vi "MH_DataToPTUTag.vi"(8 "error in":errorcluster, 10 "TagIn":T1) -> (0 "error in 2":errorcluster, 1 "AuxStrTagValue":string, 2 "TagValue":i64, 3 "TagIdent Out":string, 4 "StrTagType":string)   [LabVIEW 2019]
uses:
  <vilib>/Utility/miscctls.llb/LVDateTimeRec.ctl
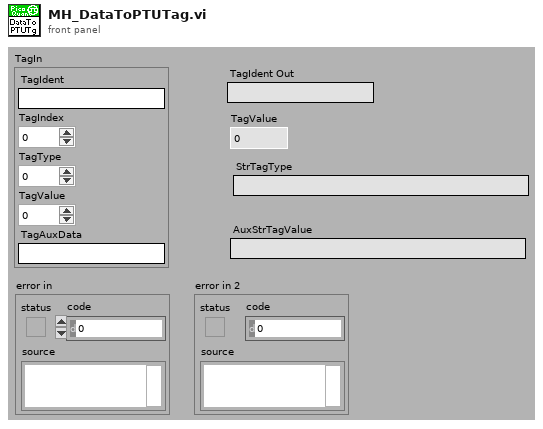
[diagram p1: front panel]
types:
  T1 = cluster{"TagIdent":string, "TagIndex":i32, "TagType":i32, "TagValue":i64, "TagAuxData":string}
  T2 = cluster{"File_GUID":string, "File_AssuredContent":string, "CreatorSW_ContentVersion":string, "CreatorSW_Name":string, "CreatorSW_Version":string, "horodatage":timestamp, "File_Comment":string}
  T3 = typedef "LVDateTimeRec.ctl" = cluster{"fractional second":dbl, "second":i32, "minute":i32, "hour":i32, "day of month":i32, "month":i32, "year":i32, "day of week":i32, "day of year":i32, "DST":i32}
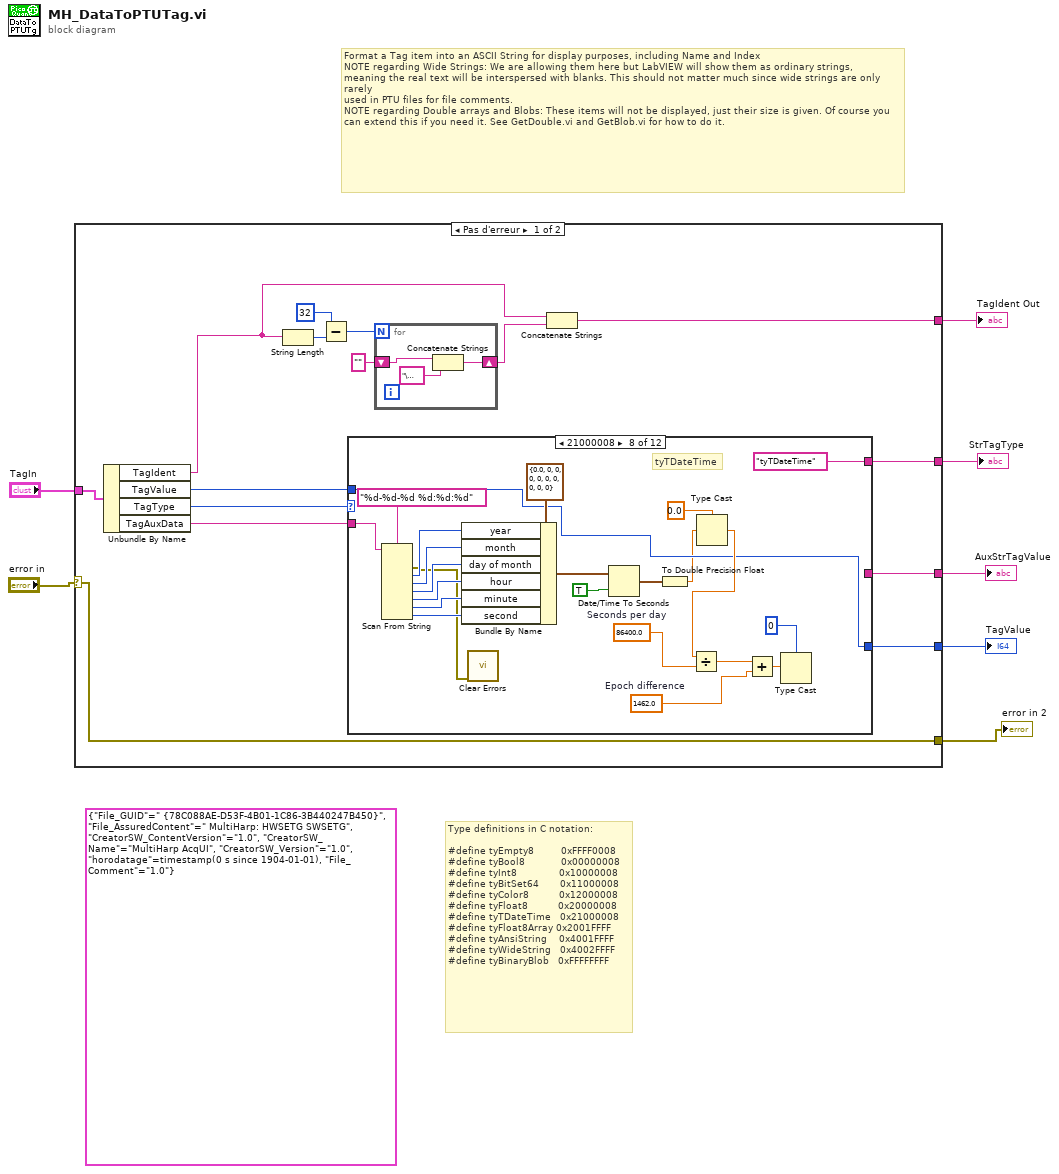
[diagram p0: block diagram]
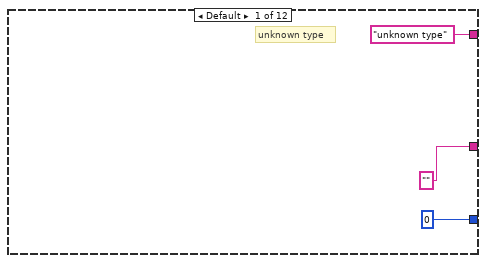
[diagram p2: hidden frame]
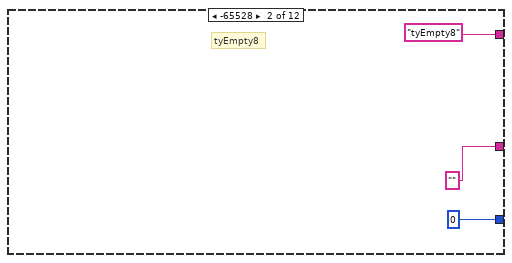
[diagram p3: hidden frame]
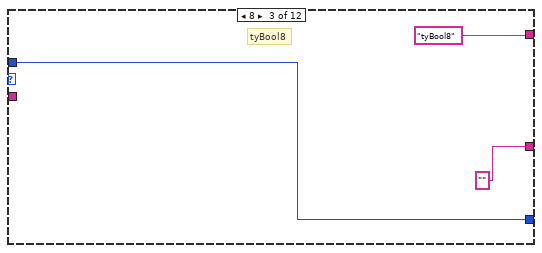
[diagram p4: hidden frame]
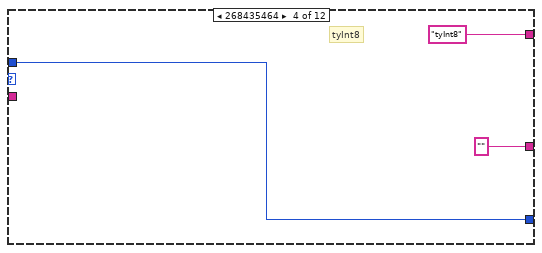
[diagram p5: hidden frame]
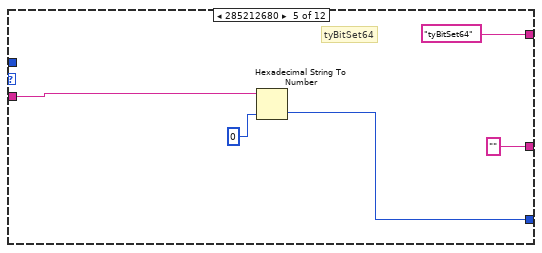
[diagram p6: hidden frame]
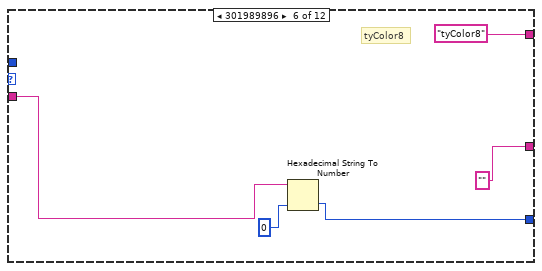
[diagram p7: hidden frame]
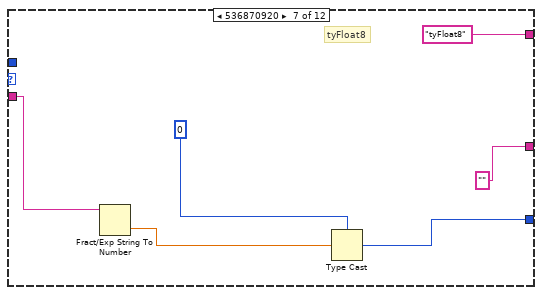
[diagram p8: hidden frame]
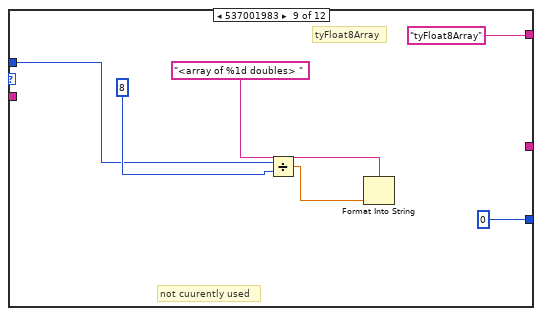
[diagram p9: hidden frame]
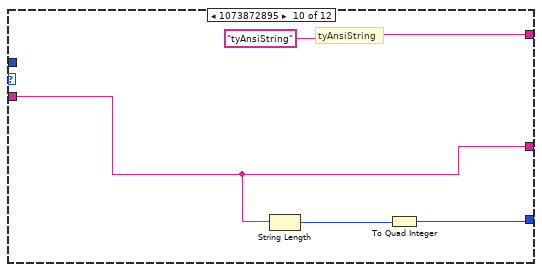
[diagram p10: hidden frame]
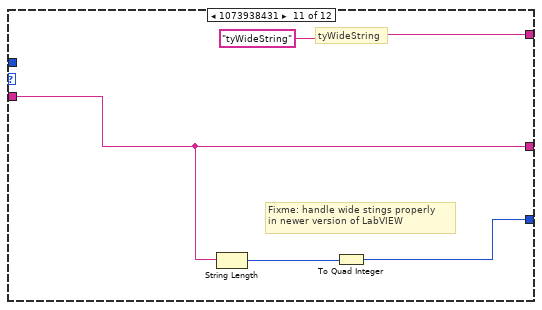
[diagram p11: hidden frame]
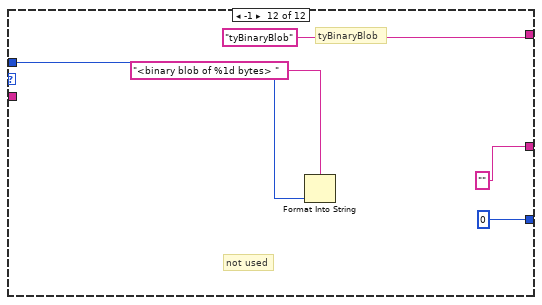
[diagram p12: hidden frame]
diagram:
  (unwired) T2 {"File_GUID"=" {78C088AE-D53F-4B01-1C86-3B440247B450}", "File_AssuredContent"=" MultiHarp: HWSETG SWSETG", "CreatorSW_ContentVersion"="1.0", "CreatorSW_Name"="MultiHarp AcqUI", "CreatorSW_Version"="1.0", "horodatage"=timestamp(0 s since 1904-01-01), "File_Comment"="1.0"}
  # "Type definitions in C notation:\n\n#define tyEmpty8         0xFFFF0008\n#define tyBool8            0x00000008\n#define tyInt8              0x10000008\n#define tyBitSet64       0x11000008\n#define tyColor8          0x12000008\n#define tyFloat8          0x20000008\n#define tyTDateTime   0x21000008\n#define tyFloat8Array 0x2001FFFF\n#define tyAnsiString    0x4001FFFF\n#define tyWideString   0x4002FFFF\n#define tyBinaryBlob   0xFFFFFFFF"
  # "Format a Tag item into an ASCII String for display purposes, including Name and Index\nNOTE regarding Wide Strings: We are allowing them here but LabVIEW will show them as ordinary strings, \nmeaning the real text will be interspersed with blanks. This should not matter much since wide strings are only rarely \nused in PTU files for file comments.\nNOTE regarding Double arrays and Blobs: These items will not be displayed, just their size is given. Of course you\ncan extend this if you need it. See GetDouble.vi and GetBlob.vi for how to do it."
  n1 = case shown="Pas d'erreur" "error in" {
    selector: "error in" -> [w10 w96]
    tunnel: [w22 _] -> w7
    tunnel: [w21 _] -> w6
    tunnel: [w16 _] -> w5
    tunnel: [w13 _] -> w4
    tunnel: "TagIn" -> [w12 _]
    tunnel: [w10 w96] -> w1
    frame No Error {
      n2 = Unbundle By Name(w12) -> ("TagIdent"=w11:string, "TagValue"=w14:i64, "TagType"=w9:i32, "TagAuxData"=w15:string)
      n3 = String Length(string=w11) -> (length=w20:i32)
      n4 = Subtract(x=32, y=w20) -> (x-y=w18:i32)
      n5 = case shown="21000008" w9 {
        tunnel: w14 -> [_ _ w32 w36 _ _ _ w55 w81 _ _ w93]
        tunnel: ["" ("TagAuxData") "" ("TagAuxData") "" ("TagAuxData") "" ("TagAuxData") "" ("TagAuxData") "" ("TagAuxData") "" ("TagAuxData") _ _ w85 w88 "" ("TagAuxData")] -> w21
        tunnel: w15 -> [_ _ _ _ w40 w45 w50 w60 _ w85 w88 _]
        tunnel: ["unknown type" ("string") "tyEmpty8" ("string") "tyBool8" ("string") "tyInt8" ("string") "tyBitSet64" ("string") "tyColor8" ("string") "tyFloat8" ("string") "tyTDateTime" ("string") "tyFloat8Array" ("string") "tyAnsiString" ("string") "tyWideString" ("string") "tyBinaryBlob" ("string")] -> w22
        tunnel: [i64 0 ("TagValue") i64 0 ("TagValue") w32 w36 w39 w44 w51 w55 i64 0 ("TagValue") w83 w87 i64 0 ("TagValue")] -> w13
        frame Default {
          # "unknown type"
        }
        frame -65528 {
          # "tyEmpty8"
        }
        frame 8 {
          # "tyBool8"
        }
        frame 268435464 {
          # "tyInt8"
        }
        frame 285212680 {
          # "tyBitSet64"
          n6 = Hexadecimal String To Number(string=w40, default (0uL)=i64 0 ("TagValue")) -> (number=w39:i64)  [unwired: 1 in, 1 out]
        }
        frame 301989896 {
          # "tyColor8"
          n7 = Hexadecimal String To Number(string=w45, default (0uL)=i64 0 ("TagValue")) -> (number=w44:i64)  [unwired: 1 in, 1 out]
        }
        frame 536870920 {
          # "tyFloat8"
          n8 = Fract/Exp String To Number(string=w50) -> (number=w49:dbl)  [unwired: 3 in, 1 out]
          n9 = Type Cast(type=i64 0 ("TagValue"), x=w49) -> (*(type *) &x=w51:i64)
        }
        frame 553648136 {
          w75 = 86400.0  # Seconds per day
          w73 = 1462.0  # Epoch difference
          # "tyTDateTime"
          n10 = Scan From String(format string="%d-%d-%d %d:%d:%d" ("chaîne de format"), input string=w60) -> (error out=w56:errorcluster, output 1=w63:i32, output 2=w64:i32, output 3=w65:i32, output 4=w66:i32, output 5=w67:i32, output 6=w68:i32)  [unwired: 8 in, 2 out]
          n11 = Bundle By Name(cluster=T3 {"fractional second"=0.0, "second"=0, "minute"=0, "hour"=0, "day of month"=0, "month"=0, "year"=0, "day of week"=0, "day of year"=0, "DST"=0} ("cluster date/heure"), "year"=w63, "month"=w64, "day of month"=w65, "hour"=w66, "minute"=w67, "second"=w68) -> (w62:T3)
          n12 = call <vilib>:"Clear Errors.vi"("error in (no error)"=w56) -> ()  [unwired: 5 in, 2 out]
          n13 = Date/Time To Seconds(1:TRUE ("UTC (F)"), 2:w62) -> (0:w59:timestamp)
          n14 = To Double Precision Float(number=w59) -> (double precision float=w54:dbl)
          n15 = Type Cast(type=0.0, x=w54) -> (*(type *) &x=w57:dbl)
          n16 = Divide(x=w57, y=w75) -> (x/y=w74:dbl)
          n17 = Add(x=w74, y=w73) -> (x+y=w72:dbl)
          n18 = Type Cast(type=i64 0 ("TagValue"), x=w72) -> ()  [unwired: 1 out]
        }
        frame 537001983 {
          # "not cuurently used"
          # "tyFloat8Array"
          n19 = Divide(x=w81, y=i64 8) -> (x/y=w80:dbl)
          n20 = Format Into String(format string="<array of %1d doubles> ", w80) -> ()  [unwired: 2 in, 2 out]
        }
        frame 1073872895 {
          # "tyAnsiString"
          n21 = String Length(string=w85) -> (length=w84:i32)
          n22 = To Quad Integer(1:w84) -> (0:w83:i64)
        }
        frame 1073938431 {
          # "Fixme: handle wide stings properly \nin newer version of LabVIEW"
          # "tyWideString"
          n23 = String Length(string=w88) -> (length=w89:i32)
          n24 = To Quad Integer(1:w89) -> (0:w87:i64)
        }
        frame -1 {
          # "not used"
          # "tyBinaryBlob"
          n25 = Format Into String(format string="<binary blob of %1d bytes> ", w93) -> ()  [unwired: 2 in, 2 out]
        }
      }
      n26 = for {
        N: w18 -> [_]
        shift-right: [w25] -> w17
        shift-left: "" -> [w24]
        n27 = Concatenate Strings(w24, "\u0000") -> (w25:string)
      }
      n28 = Concatenate Strings(w11, w17) -> (w16:string)
    }
    frame Error {
    }
  }
  "StrTagType" <- w7
  "AuxStrTagValue" <- w6
  "TagIdent Out" <- w5
  "TagValue" <- w4
  "error in 2" <- w1
